vi "Connect.vi"(8 "error in (no error)":errorcluster, 11 "Bluetooth Address":string) -> (0 "error out":errorcluster, 3 "Output data":refnum<k31>)   [LabVIEW 2014]
doc: "Initializes a bluetooth connection in the specified adapter"
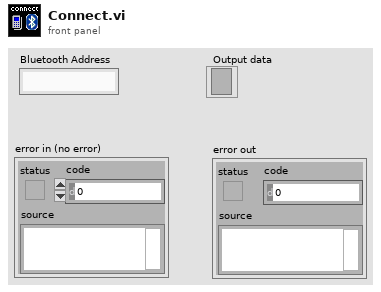
[diagram p1: front panel]
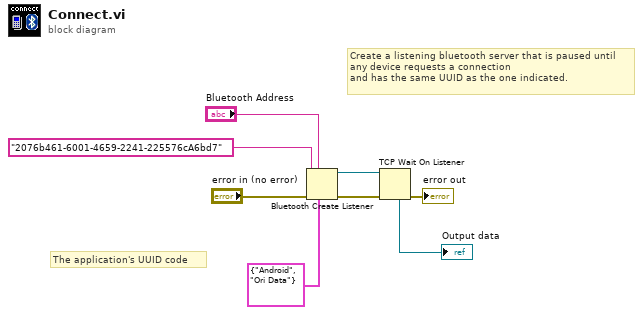
[diagram p0: block diagram]
diagram:
  # "Create a listening bluetooth server that is paused until\nany device requests a connection \nand has the same UUID as the one indicated."
  # "The application's UUID code"
  n1 = Bluetooth Create Listener(6:cluster{"name":string, "description":string} {"name"="Android", "description"="Ori Data"} ("service description"), 7:"Bluetooth Address", 8:"error in (no error)", 10:"2076b461-6001-4659-2241-225576cA6bd7" ("uuid")) -> (0:w5:errorcluster, 3:w6:refnum<k31>)  [unwired: 1 out]
  n2 = TCP Wait On Listener(8:w5, 11:w6) -> (0:→"error out":errorcluster, 4:→"Output data":refnum<k31>)  [unwired: 5 out]
